vi "robust state change detection.vi"(7 "falling edge (F)":bool, 8 "history":bool[](array[boolean]), 9 "step":i16, 10 "tick":i32, 11 "New state":bool) -> (0 "history out":bool[](array[boolean]), 1 "step out":i16, 2 "edge detected":bool, 3 "Stop?":bool, 4 "tick":u32)   [LabVIEW 2018]
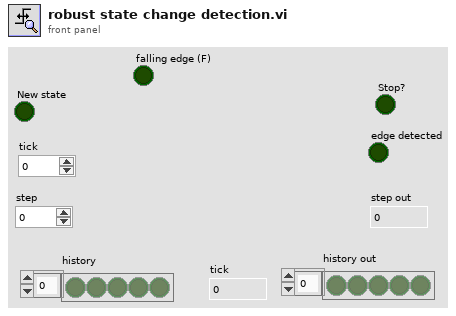
[diagram p1: front panel]
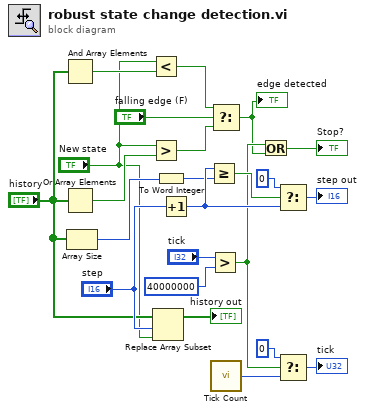
[diagram p0: block diagram]
diagram:
  n1 = And Array Elements(Boolean array="history") -> (logical AND=w7:bool)
  n2 = Or Array Elements(Boolean array="history") -> (logical OR=w8:bool)
  n3 = Array Size(array="history") -> (size(s)=w10:i32)
  n4 = Less?(x="New state", y=w7) -> (x < y?=w6:bool)
  n5 = Greater?(x="New state", y=w8) -> (0:w5:bool)
  n6 = Replace Array Subset(array="history", new element="New state", index="step") -> (→"history out":bool[])
  n7 = To Word Integer(number=w10) -> (16bit integer=w9:i16)
  n8 = Increment(x="step") -> (x+1=w15:i16)
  n9 = Greater Or Equal?(x=w15, y=w9) -> (x >= y?=w16:bool)
  n10 = Greater?(x="tick", y=40000000) -> (0:w12:bool)
  n11 = Select(t=w6, s="falling edge (F)", f=w5) -> (s? t:f=w1:bool)
  "edge detected" <- w1
  n12 = call "Tick Count"() -> ("Tick Count(Ticks)"=w21:u32)
  n13 = Or(x=w12, y=w1) -> (x .or. y?=→"Stop?":bool)
  n14 = Select(t=i16 0, s=w16, f=w15) -> (s? t:f=→"step out":i16)
  n15 = Select(t=u32 0, s=w12, f=w21) -> (s? t:f=→"tick":u32)
